vi "0037-Sub_map2.vi"(7 "error out":errorcluster, 9 "アドレス":i32, 10 "device":T2) -> (0 "error out 2":errorcluster caption="error out", 1 "x = y?":bool, 3 "device 2":T2)   [LabVIEW 2014]
uses:
  LV-CP2112_2014/LVProject/private/CP2112_device.ctl
  LV-CP2112_2014/LVProject/private/CP2112_SMBUS_S0.ctl
panel:
  out "HID_SMBUS_S0":T1
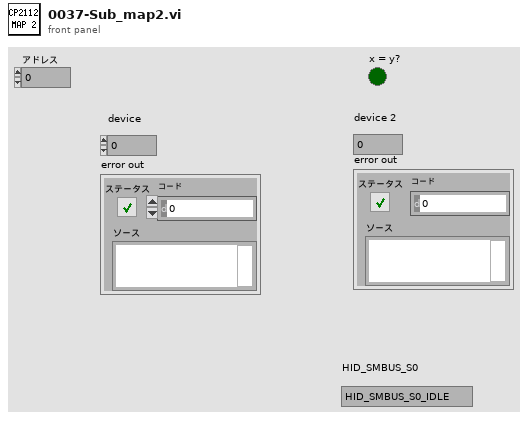
[diagram p1: front panel]
types:
  T1 = typedef "CP2112_SMBUS_S0.ctl" = enum8{"HID_SMBUS_S0_IDLE", "HID_SMBUS_S0_BUSY", "HID_SMBUS_S0_COMPLETE", "HID_SMBUS_S0_ERROR"}
  T2 = typedef "CP2112_device.ctl" = i32
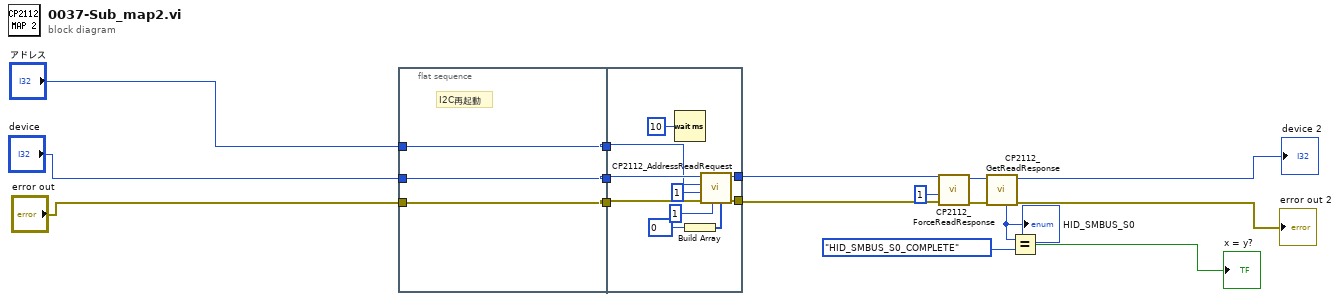
[diagram p0: block diagram]
diagram:
  n1 = flat-sequence {
    tunnel: "device" -> [w18]
    tunnel: "error out" -> [w19]
    tunnel: "アドレス" -> [w17]
    tunnel: [w18] -> w10
    tunnel: [w19] -> w9
    tunnel: [w17] -> w8
    tunnel: w10 -> [w25]
    tunnel: w9 -> [w26]
    tunnel: w8 -> [w24]
    tunnel: [w22] -> w7
    tunnel: [w21] -> w6
    frame #0 {
      # "I2C再起動"
    }
    frame #1 {
      n2 = Wait (ms)(milliseconds to wait=u32 10 ("ミリ秒待機時間")) -> ()  [unwired: 1 out]
      n3 = Build Array(u8 0 ("targetAddressSize")) -> (w20:u8[])
      n4 = call "CP2112_AddressReadRequest.vi"("targetAddress[]"=w20, "targetAddressSize"=u8 1, "error in (no error)"=w26, "numByteToRead"=i16 1, "slaveAddress"=w24, "device"=w25) -> ("error out"=w22:errorcluster, "deviceOut"=w21:T2)  [unwired: 3 in, 1 out]
    }
  }
  n5 = call "CP2112_ForceReadResponse.vi"("error in (no error)"=w7, "numByteToRead"=i16 1, "device"=w6) -> ("error out"=w16:errorcluster, "deviceOut"=w15:T2)  [unwired: 6 in, 1 out]
  n6 = call "CP2112_GetReadResponse.vi"("error in (no error)"=w16, "device"=w15) -> ("error out"=→"error out 2":errorcluster, "deviceOut"=→"device 2":T2, "HID_SMBUS_S0"=w12:T1)  [unwired: 4 in, 3 out]
  "HID_SMBUS_S0" <- w12
  n7 = Equal?(x=w12, y=CP2112_SMBUS_S0."HID_SMBUS_S0_COMPLETE" ("HID_SMBUS_S0")) -> (x = y?=→"x = y?":bool)
